vi "chart legend delete series.vi"(8 "error in (no error)":errorcluster, 10 "delete_series":u32, 11 "chart":u32) -> (0 "error out":errorcluster, 3 "function return":u32(ring))   [LabVIEW 8.6]
doc: "lxw_error chart_legend_delete_series(lxw_chart chart, unsigned long delete_series);"
uses:
  pending_lvxlsxwriter/xlsxwriter.dll
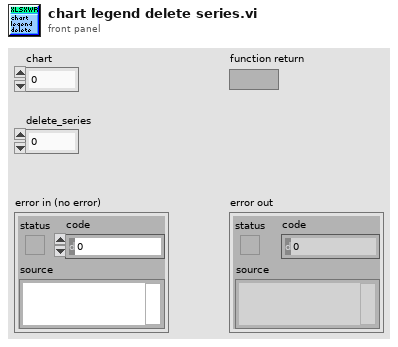
[diagram p1: front panel]
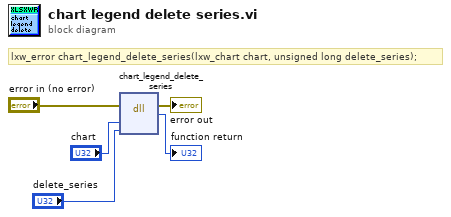
[diagram p0: block diagram]
diagram:
  # "lxw_error chart_legend_delete_series(lxw_chart chart, unsigned long delete_series);"
  n1 = dll-call lib="C:/Users/WDAGUtilityAccount/Desktop/pending_lvxlsxwriter/xlsxwriter.*" fn="chart_legend_delete_series"(error in="error in (no error)", "chart"="chart", "delete_series"="delete_series") -> (error out=→"error out":errorcluster, →"function return":u32)  [unwired: 4 in, 1 out]
